vi "Player Info.vi"(11 "Expand in":refnum<class "Expand.lvclass">) -> (1 "Victory Speech":string, 2 "Name":string, 3 "Expand out":refnum<class "Expand.lvclass">)   [LabVIEW 2015, in "Expand.lvclass"]
uses:
  Expand.lvclass
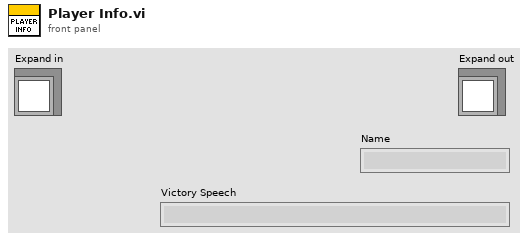
[diagram p1: front panel]
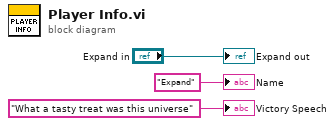
[diagram p0: block diagram]
diagram:
  "Expand out" <- "Expand in"
  "Name" <- "Expand" ("Name")
  "Victory Speech" <- "What a tasty treat was this universe" ("Victory Speech")
